vi "FormatDateTime.vi"(8 "error in":errorcluster, 10 "Unformatted  Date":timestamp) -> (0 "error out":errorcluster, 1 "Time":string, 2 "Date":string)   [LabVIEW 2020]
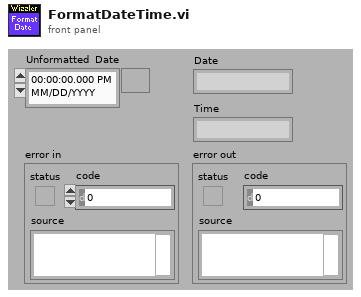
[diagram p1: front panel]
types:
  T1 = typedef "LVDateTimeRec.ctl" = cluster{"fractional second":dbl, "second":i32, "minute":i32, "hour":i32, "day of month":i32, "month":i32, "year":i32, "day of week":i32, "day of year":i32, "DST":i32}
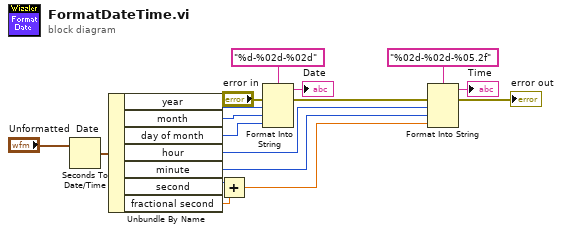
[diagram p0: block diagram]
diagram:
  n1 = Seconds To Date/Time(time stamp (now)="Unformatted  Date") -> (date time rec=w17:T1)  [unwired: 1 in]
  n2 = Unbundle By Name(w17) -> ("year"=w15:i32, "month"=w14:i32, "day of month"=w13:i32, "hour"=w11:i32, "minute"=w10:i32, "second"=w9:i32, "fractional second"=w7:dbl)
  n3 = Add(x=w9, y=w7) -> (x+y=w8:dbl)
  n4 = Format Into String(format string="%d-%02d-%02d", error in="error in", w15, w14, w13) -> (resulting string=→"Date":string, error out=w6:errorcluster)  [unwired: 1 in]
  n5 = Format Into String(format string="%02d-%02d-%05.2f", error in=w6, w11, w10, w8) -> (resulting string=→"Time":string, error out=→"error out":errorcluster)  [unwired: 1 in]
